vi "IBM4_Read(IN).vi"(8 "error in":errorcluster, 9 "Number":i32=10 min=1, 10 "Channel":enum16{"A2", "A3", "A4", "A5"}(ring), 11 "COM resource in":refnum<visa-resource-name>="ASRL5::INSTR") -> (0 "error out":errorcluster, 2 "array":i32[](array[numeric]), 3 "COM resource out":refnum<visa-resource-name>="ASRL5::INSTR")   [LabVIEW 2021, in "IBM4.lvlib"]
doc: "This VI interfaces with the IBM4 to perform a read operation.\n\nThe number of readings should be greater than zero. At some point the number of reading will be too high and will cause a timeout error. This should only happen for numbers larger than 10000. The output will be an array of integer values.\n\nAlternate read operations exist covering binary or floating point, single reading, multiple readings, and an average of multiple readings (floating point only)."
uses:
  <instrlib>/IBM4/IBM4.lvlib
panel:
  out "read buffer":string="Output 3 = 1.85786 \r\n"
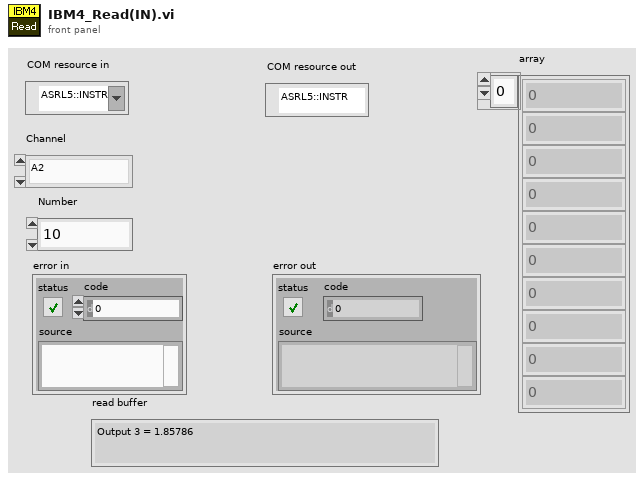
[diagram p1: front panel]
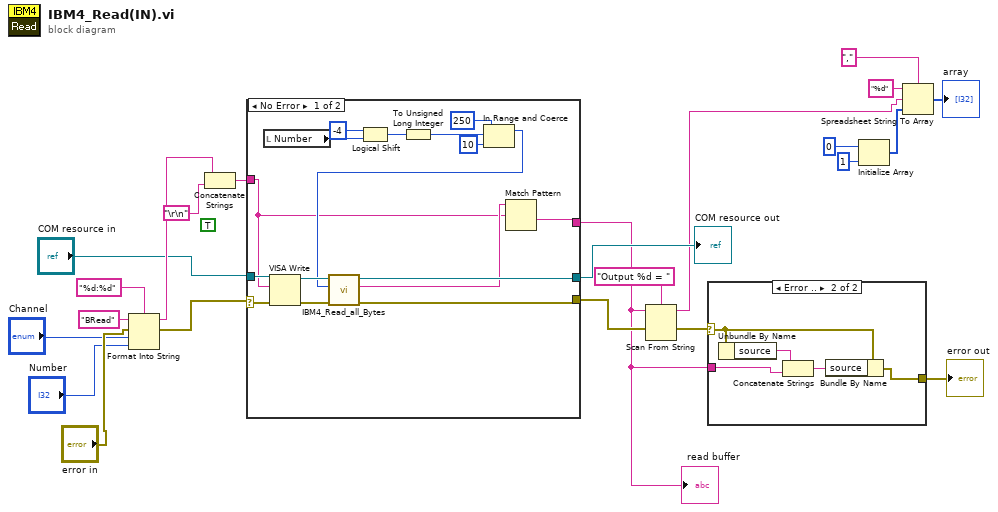
[diagram p0: block diagram]
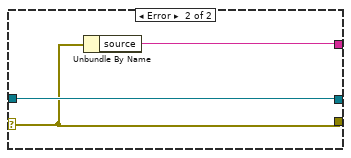
[diagram p3: hidden frame]
diagram:
  (unwired) TRUE ("Enable Termination\nChar (T)")
  n1 = Format Into String(format string="%d:%d", initial string="BRead", error in="error in", "Channel", "Number") -> (resulting string=w15:string, error out=w2:errorcluster)
  n2 = Concatenate Strings(w15, "\r\n") -> (w14:string)
  n3 = case shown="No Error" w2 {
    selector: w2 -> [w38 w40]
    tunnel: "COM resource in" -> [w39 w42]
    tunnel: [w27 w40] -> w18
    tunnel: [w26 w41] -> w11
    tunnel: w14 -> [w24 _]
    tunnel: [w28 w42] -> w19
    frame No Error {
      n4 = local read "Number"() -> (w34:i32)
      n5 = VISA Write(VISA resource name=w39, write buffer=w24, error in (no error)=w38) -> (VISA resource name out=w31:refnum<visa-resource-name>, error out=w30:errorcluster)  [unwired: 1 out]
      n6 = Logical Shift(y=i16 -4, x=w34) -> (x << y=w35:i32)
      n7 = To Unsigned Long Integer(number=w35) -> (unsigned 32bit integer=w32:u32)
      n8 = In Range and Coerce(upper limit=u32 250, x=w32, lower limit=u32 10) -> (coerced(x)=w29:u32)  [unwired: 1 out]
      n9 = call <instrlib>:"IBM4_Read_all_Bytes.vi"("error in (no error)"=w30, "milliseconds to wait"=w29, "VISA Refnum in"=w31) -> ("error out"=w27:errorcluster, "String"=w25:string, "VISA Refnum out"=w28:refnum<visa-resource-name>)  [unwired: 2 in]
      n10 = Match Pattern(string=w25, regular expression=w24) -> (after substring=w26:string)  [unwired: 1 in, 3 out]
    }
    frame Error {
      n11 = Unbundle By Name(w40) -> ("source"=w41:string)
    }
  }
  "COM resource out" <- w19
  "read buffer" <- w11
  n12 = Scan From String(format string="Output %d = ", input string=w11, error in=w18) -> (remaining string=w5:string, error out=w13:errorcluster)  [unwired: 3 in, 1 out]
  n13 = case shown="Error .." w13 {
    selector: w13 -> [w43 w47]
    tunnel: [w43 w48] -> w12
    tunnel: w11 -> [_ w44]
    frame No Error {
    }
    frame Error {
      n14 = Unbundle By Name(w47) -> ("source"=w45:string)
      n15 = Concatenate Strings(w45, w44) -> (w46:string)
      n16 = Bundle By Name(cluster=w47, "source"=w46) -> (w48:errorcluster)
    }
  }
  "error out" <- w12
  n17 = Initialize Array(0, 1 ("dimension size")) -> (w9:i32[])
  n18 = Spreadsheet String To Array(delimiter (Tab)=",", format string="%d", spreadsheet string=w5, array type (2D Dbl)=w9) -> (array=→"array":i32[])
